vi "BCU参数读取-Auto.vi"(8 "CAN端口":u16(ring), 9 "设备索引号":u16(ring), 10 "CAN卡类型":u32(ring)=21, 11 "Myindex":dbl=1.0) -> (3 "成功":bool)   [LabVIEW 2013] (continued)
                    n501 = Greater Or Equal?(x=w675, y=30) -> (x >= y?=w673:bool)
                    n502 = Wait Until Next ms Multiple(millisecond multiple=u32 100 ("毫秒倍数")) -> ()  [unwired: 1 out]
                    n503 = Compound Arithmetic op=OR(w669, w670, w673) -> (w672:bool)
                  }
                }
                frame #4 {
                  n504 = call <vilib>:"Unset Busy.vi"() -> ()  [unwired: 2 in, 10 out]
                  n505 = case shown="假" w677 {
                    tunnel: w676 -> [w678 _]
                    frame False {
                      n506 = control-ref of="结果"() -> (w682:refnum<vi>)
                      n507 = Concatenate Strings(w678, "       写入失败" ("字符串")) -> (w681:string)
                      n508 = Build Array(w681) -> (w680:string[])
                      n509 = call "表格编辑.vi"("新元素/子数组"=w680, "活动单元格:单元格背景色"=u32 16740749, "MCListbox引用句柄"=w682) -> ()  [unwired: 9 out]
                    }
                    frame True {
                    }
                  }
                }
                frame #5 {
                  n510 = Increment(x=w688) -> (x+1=w684:i32)
                  n511 = Equal?(x=w689, y=w684) -> (x = y?=w687:bool)
                  n512 = And(x=w686, y=w687) -> (x .and. y?=w685:bool)
                  n513 = case shown="真" w685 {
                    frame False {
                    }
                    frame True {
                      n514 = control-ref of="结果"() -> (w693:refnum<vi>)
                      n515 = Concatenate Strings("写入完成" ("字符串")) -> (w692:string)
                      n516 = Build Array(w692) -> (w691:string[])
                      n517 = call "表格编辑.vi"("新元素/子数组"=w691, "活动单元格:单元格背景色"=u32 21937, "MCListbox引用句柄"=w693) -> ()  [unwired: 9 out]
                    }
                  }
                }
              }
            }
            n518 = local read "强制终止读写标记"() -> (w586:bool)
            n519 = Or(x=w584, y=w586) -> (x .or. y?=w585:bool)
          }
          n520 = stacked-sequence {
            tunnel: w576 -> [_]
            frame #0 {
              n521 = call <vilib>:"Unset Busy.vi"() -> ()  [unwired: 2 in, 10 out]
              n522 = local write "强制终止读写标记"(FALSE ("强制停止")) -> ()
            }
          }
        }
        frame "单个读取" {
          n523 = stacked-sequence {
            tunnel: [w726] -> w724
            frame #0 {
              n524 = local read "主从选择"() -> (w727:enum32{"主板", "从板"})
              n525 = case shown="\"主板\", 默认" w727 {
                tunnel: [w740 w823] -> w729
                tunnel: [w739 w824] -> w734
                tunnel: [0 ("从板号") w820] -> w733
                tunnel: [0 ("板号") u8 0 ("板号")] -> w732
                tunnel: [w735 w819] -> w730
                frame "主板", Default {
                  n526 = local read "主板选项"() -> (w736:string)
                  n527 = case shown="\"二维码\"" w736 {
                    tunnel: [_ u8[] [1, 2, 3, 4, 5, 6, 13, 8, 7, 9, 10, 11, 12] u8[] [1] u8[] [1] u8[] [1] u8[] [2] u8[] [3] u8[] [4] u8[] [5] u8[] [6] u8[] [13] u8[] [7] u8[] [8] u8[] [9] u8[] [10] u8[] [14] u8[] [11] u8[] [12] u8[] [2] u8[] [3] u8[] [1] u8[] [2] u8[] [1] u8[] [2] u8[] [3] u8[] [4] u8[] [1, 2, 3, 4]] -> w740
                    tunnel: [_ u8 128 ("命令") u8 129 ("命令") u8 128 ("命令") u8 140 ("命令") u8 128 ("命令") u8 128 ("命令") u8 128 ("命令") u8 128 ("命令") u8 128 ("命令") u8 128 ("命令") u8 128 ("命令") u8 128 ("命令") u8 128 ("命令") u8 128 ("命令") u8 128 ("命令") u8 128 ("命令") u8 128 ("命令") u8 129 ("命令") u8 129 ("命令") u8 130 ("命令") u8 130 ("命令") u8 132 ("命令") u8 132 ("命令") u8 132 ("命令") u8 132 ("命令") u8 132 ("命令")] -> w739
                    tunnel: [_ string[] ["产品编号", "电压个数", "通道电压数", "电压起始值", "温度个数", "温度起始值", "保险位置", "电池额定实际容量", "SOC", "配置文件版本", "参数修改记录", "车牌号", "SOH"] string[] ["一级故障阀值"] string[] ["产品编号"] string[] ["读二维码"] string[] ["电压个数"] string[] ["通道电压数"] string[] ["电压起始值"] string[] ["温度个数"] string[] ["温度起始值"] string[] ["保险位置"] string[] ["SOC"] string[] ["电池额定实际容量"] string[] ["配置文件版本"] string[] ["参数修改记录"] string[] ["校正时钟"] string[] ["车牌号"] string[] ["SOH"] string[] ["二级故障阀值"] string[] ["三级故障阀值"] string[] ["加热控制参数"] string[] ["充电控制参数"] string[] ["电池信息1"] string[] ["电池包组号"] string[] ["充放电安时"] string[] ["电池充放电次数"] string[] ["电池信息1", "电池包组号", "充放电安时", "电池充放电次数"]] -> w735
                    frame "假", Default {
                    }
                    frame "项目信息" {
                    }
                    frame "SOC过低", "SOC过高", "SOH过低", "充电电流过高", "单体电压过低", "单体电压过高", "单组电压不均衡", "单组温度不均衡", "放电电流过高", "极柱温度过高", "内阻过大", "温度过低", "温度过高", "一级故障阀值", "整组电压不均衡", "整组温度不均衡", "总电压过低", "总电压过高" {
                    }
                    frame "产品编号" {
                    }
                    frame "二维码" {
                    }
                    frame "电压个数" {
                    }
                    frame "通道电压数" {
                    }
                    frame "电压起始值" {
                    }
                    frame "温度个数" {
                    }
                    frame "温度起始值" {
                    }
                    frame "保险位置" {
                    }
                    frame "SOC" {
                    }
                    frame "电池额定实际容量" {
                    }
                    frame "配置文件版本" {
                    }
                    frame "参数修改记录" {
                    }
                    frame "校正时钟" {
                    }
                    frame "车牌号" {
                    }
                    frame "SOH" {
                    }
                    frame "SOC过低(2)", "SOC过高(2)", "SOH过低(2)", "充电电流过高(2)", "单体电压过低(2)", "单体电压过高(2)", "单组电压不均衡(2)", "单组温度不均衡(2)", "二级故障阀值", "放电电流过高(2)", "极柱温度过高(2)", "内阻过大(2)", "温度过低(2)", "温度过高(2)", "整组电压不均衡(2)", "整组温度不均衡(2)", "总电压过低(2)", "总电压过高(2)" {
                    }
                    frame "SOC过低(3)", "SOC过高(3)", "SOH过低(3)", "充电电流过高(3)", "单体电压过低(3)", "单体电压过高(3)", "单组电压不均衡(3)", "单组温度不均衡(3)", "放电电流过高(3)", "极柱温度过高(3)", "内阻过大(3)", "三级故障阀值", "温度过低(3)", "温度过高(3)", "整组电压不均衡(3)", "整组温度不均衡(3)", "总电压过低(3)", "总电压过高(3)" {
                    }
                    frame "风机关闭温差", "风机关闭温度", "风机开启温差", "风机开启温度", "加热关闭温差", "加热关闭温度", "加热开启温度", "加热控制参数" {
                    }
                    frame "充电控制参数", "电流步长", "最大允许充电电流", "最大允许充电温度", "最大允许单体电压", "最大允许总电压", "最小允许充电电流", "最小允许充电温度", "最小允许单体电压" {
                    }
                    frame "电池信息1" {
                    }
                    frame "电池包组号" {
                    }
                    frame "充放电安时" {
                    }
                    frame "电池充放电次数" {
                    }
                    frame "电池信息" {
                    }
                  }
                }
                frame "从板" {
                  n528 = local read "从板选项"() -> (w821:string)
                  n529 = case shown="\"二维码\"" w821 {
                    tunnel: [_ u8 0 ("命令") u8 10 ("命令") u8 0 ("命令") u8 0 ("命令") u8 0 ("命令") u8 0 ("命令") u8 0 ("命令") u8 0 ("命令") u8 2 ("命令") u8 2 ("命令") u8 2 ("命令") u8 3 ("命令") u8 6 ("命令") u8 6 ("命令") u8 6 ("命令") u8 3 ("命令") u8 3 ("命令") u8 3 ("命令") u8 3 ("命令") u8 3 ("命令") u8 3 ("命令") u8 3 ("命令")] -> w824
                    tunnel: [_ u8[] [6] u8[] [1] u8[] [6, 1, 2, 3, 4, 5] u8[] [1] u8[] [2] u8[] [3] u8[] [4] u8[] [5] u8[] [1] u8[] [2] u8[] [3] u8[] [1, 2, 3, 4, 5, 6, 7] u8[] [1, 2] u8[] [2] u8[] [1] u8[] [1] u8[] [2] u8[] [3] u8[] [4] u8[] [5] u8[] [6] u8[] [7]] -> w823
                    tunnel: [_ string[] ["从板号"] string[] ["读二维码"] string[] ["从板号", "电压起始值", "通道电压个数", "保险位置", "温度起始值", "加热控制参数"] string[] ["电压起始值"] string[] ["通道电压节数"] string[] ["保险位置"] string[] ["温度起始值"] string[] ["加热控制参数"] string[] ["一级故障阀值"] string[] ["二级故障阀值"] string[] ["三级故障阀值"] string[] ["电池包信息1", "电池包序号", "充放电安时", "充电次数时间", "SOC", "车牌号", "充电参数"] string[] ["均衡阀值", "充电结束电压"] string[] ["充电结束电压"] string[] ["均衡阀值"] string[] ["电池包信息1"] string[] ["电池包序号"] string[] ["充放电安时"] string[] ["充电次数时间"] string[] ["SOC"] string[] ["车牌号"] string[] ["充电参数"]] -> w819
                    frame "假", Default {
                    }
                    frame "从板号" {
                    }
                    frame "二维码" {
                    }
                    frame "从板信息" {
                    }
                    frame "电压个数" {
                    }
                    frame "通道电压节数" {
                    }
                    frame "保险位置" {
                    }
                    frame "温度个数" {
                    }
                    frame "风机关闭温差", "风机关闭温度", "风机开启温差", "风机开启温度", "加热关闭温差", "加热关闭温度", "加热开启温度", "加热控制参数" {
                    }
                    frame "SOC过低", "电压不均衡", "电压过低", "电压过高", "温度不均衡", "温度过低", "温度过高", "一级故障阀值" {
                    }
                    frame "SOC过低(2)", "电压不均衡(2)", "电压过低(2)", "电压过高(2)", "二级故障阀值", "温度不均衡(2)", "温度过低(2)", "温度过高(2)" {
                    }
                    frame "SOC过低(3)", "电压不均衡(3)", "电压过低(3)", "电压过高(3)", "三级故障阀值", "温度不均衡(3)", "温度过低(3)", "温度过高(3)" {
                    }
                    frame "快换参数" {
                    }
                    frame "均衡参数" {
                    }
                    frame "充电结束电压" {
                    }
                    frame "均衡阀值" {
                    }
                    frame "电池包信息1" {
                    }
                    frame "电池包序号" {
                    }
                    frame "充放电安时" {
                    }
                    frame "充电次数时间" {
                    }
                    frame "SOC" {
                    }
                    frame "车牌号" {
                    }
                    frame "充电参数" {
                    }
                  }
                  n530 = local read "从板号"() -> (w820:u8)
                }
              }
              n531 = Build Array(w732) -> (w731:i32[])
              n532 = local write "命令"(w734) -> ()
              n533 = Array Size(array=w729) -> (size(s)=w728:i32)
              n534 = for {
                tunnel: w729 -> [w899] mode=indexing
                tunnel: w734 -> [w898]
                tunnel: w733 -> [w897]
                tunnel: w731 -> [w896]
                tunnel: w730 -> [w895] mode=indexing
                tunnel: w728 -> [w894]
                tunnel: w727 -> [w892]
                tunnel: [w891] -> w726
                i -> [w893]
                n535 = while {
                  tunnel: w899 -> [w908]
                  tunnel: w898 -> [w907]
                  tunnel: w897 -> [w906]
                  tunnel: w896 -> [w905]
                  tunnel: w895 -> [w904]
                  tunnel: w894 -> [w903]
                  tunnel: w893 -> [w902]
                  tunnel: w892 -> [w901]
                  tunnel: [w900] -> w891
                  stop <- w900 stop-if-true
                  n536 = stacked-sequence {
                    seq-local: [_ _ _ _ w1058 _ _] -> [_ _ _ _ _ w1067 _]
                    tunnel: w908 -> [_ _ _ w1046 _ _ _]
                    tunnel: w907 -> [_ _ _ w1045 _ _ _]
                    tunnel: w906 -> [_ _ _ w1044 _ _ _]
                    tunnel: w905 -> [_ _ _ w1043 _ _ _]
                    tunnel: [_ _ _ _ w1059 _ _] -> w900
                    tunnel: w904 -> [w910 _ _ _ _ w1068 _]
                    tunnel: w903 -> [_ _ _ _ _ _ w1078]
                    tunnel: w902 -> [_ _ _ _ _ _ w1077]
                    tunnel: w901 -> [w909 _ _ _ _ _ _]
                    frame #0 {
                      n537 = case shown="\"从板\"" w909 {
                        tunnel: w910 -> [w911 w1003]
                        frame "主板", Default {
                          n538 = case shown="\"读二维码\"" w911 {
                            frame "假", Default {
                            }
                            frame "产品编号" {
                              n539 = control-ref of="产品编号"() -> (w913:refnum<vi>)
                              n540 = property class="Str"(reference=w913, "Value"="") -> ()  [unwired: 1 in, 2 out]
                            }
                            frame "读二维码" {
                              n541 = local write "二维码信息"("" ("二维码信息")) -> ()
                            }
                            frame "电压个数" {
                              n542 = local read "从板个数"() -> (w915:dbl)
                              n543 = control-ref of="项目信息"() -> (w919:refnum<vi>)
                              n544 = for {
                                N: w915 -> [_]
                                tunnel: [""] -> w918 mode=indexing
                              }
                              n545 = call "表格数据输入-8.6.vi"("行数"=u32 0, "列数"=u32 1, "字符串数组"=w918, "表格引用"=w919) -> ()  [unwired: 8 in]
                            }
                            frame "通道电压数" {
                              n546 = control-ref of="项目信息"() -> (w925:refnum<vi>)
                              n547 = for {
                                N: 20 -> [_]
                                tunnel: [""] -> w924 mode=indexing
                              }
                              n548 = local read "从板个数"() -> (w926:dbl)
                              n549 = Increment(x=w926) -> (x+1=w922:dbl)
                              n550 = call "表格数据输入-8.6.vi"("行数"=w922, "列数"=u32 1, "字符串数组"=w924, "表格引用"=w925) -> ()  [unwired: 8 in]
                            }
                            frame "电压起始值" {
                              n551 = local read "从板个数"() -> (w930:dbl)
                              n552 = Increment(x=w930) -> (x+1=w929:dbl)
                              n553 = control-ref of="项目信息"() -> (w936:refnum<vi>)
                              n554 = for {
                                N: w929 -> [_]
                                tunnel: [""] -> w935 mode=indexing
                              }
                              n555 = Multiply(x=u8 1, y=w930) -> (x*y=w932:dbl)
                              n556 = Add(x=w932, y=u8 21) -> (x+y=w928:dbl)
                              n557 = call "表格数据输入-8.6.vi"("行数"=w928, "列数"=u32 1, "字符串数组"=w935, "表格引用"=w936) -> ()  [unwired: 8 in]
                            }
                            frame "温度个数" {
                              n558 = local read "从板个数"() -> (w940:dbl)
                              n559 = Increment(x=w940) -> (x+1=w939:dbl)
                              n560 = control-ref of="项目信息"() -> (w946:refnum<vi>)
                              n561 = for {
                                N: w939 -> [_]
                                tunnel: [""] -> w945 mode=indexing
                              }
                              n562 = Multiply(x=u8 2, y=w940) -> (x*y=w942:dbl)
                              n563 = Add(x=w942, y=u8 22) -> (x+y=w938:dbl)
                              n564 = call "表格数据输入-8.6.vi"("行数"=w938, "列数"=u32 1, "字符串数组"=w945, "表格引用"=w946) -> ()  [unwired: 8 in]
                            }
                            frame "温度起始值" {
                              n565 = local read "从板个数"() -> (w950:dbl)
                              n566 = Increment(x=w950) -> (x+1=w949:dbl)
                              n567 = control-ref of="项目信息"() -> (w956:refnum<vi>)
                              n568 = for {
                                N: w949 -> [_]
                                tunnel: [""] -> w955 mode=indexing
                              }
                              n569 = Multiply(x=u8 3, y=w950) -> (x*y=w952:dbl)
                              n570 = Add(x=w952, y=u8 23) -> (x+y=w948:dbl)
                              n571 = call "表格数据输入-8.6.vi"("行数"=w948, "列数"=u32 1, "字符串数组"=w955, "表格引用"=w956) -> ()  [unwired: 8 in]
                            }
                            frame "保险位置" {
                              n572 = local read "从板个数"() -> (w960:dbl)
                              n573 = control-ref of="项目信息"() -> (w966:refnum<vi>)
                              n574 = for {
                                N: 10 -> [_]
                                tunnel: [""] -> w965 mode=indexing
                              }
                              n575 = Multiply(x=u8 4, y=w960) -> (x*y=w962:dbl)
                              n576 = Add(x=w962, y=u8 24) -> (x+y=w959:dbl)
                              n577 = call "表格数据输入-8.6.vi"("行数"=w959, "列数"=u32 1, "字符串数组"=w965, "表格引用"=w966) -> ()  [unwired: 8 in]
                            }
                            frame "电池额定实际容量" {
                              w968 = 0.0 ("值")
                              n578 = control-ref of="电池实际容量(A)"() -> (w969:refnum<vi>)
                              n579 = control-ref of="电池额定容量(A)"() -> (w970:refnum<vi>)
                              n580 = property class="DigNum (严格)"(reference=w969, "Value"=w968) -> ()  [unwired: 1 in, 2 out]
                              n581 = property class="DigNum (严格)"(reference=w970, "Value"=w968) -> ()  [unwired: 1 in, 2 out]
                            }
                            frame "SOC" {
                              n582 = control-ref of="SOC(%)"() -> (w971:refnum<vi>)
                              n583 = property class="DigNum (严格)"(reference=w971, "Value"=0.0 ("值")) -> ()  [unwired: 1 in, 2 out]
                            }
                            frame "配置文件版本" {
                              n584 = control-ref of="配置文件版本"() -> (w973:refnum<vi>)
                              n585 = property class="Str"(reference=w973, "Value"="" ("值")) -> ()  [unwired: 1 in, 2 out]
                            }
                            frame "参数修改记录" {
                              n586 = control-ref of="使用者"() -> (w976:refnum<vi>)
                              n587 = control-ref of="系统时钟"() -> (w977:refnum<vi>)
                              n588 = property class="DigNum (严格)"(reference=w976, "Value"=0.0 ("值")) -> ()  [unwired: 1 in, 2 out]
                              n589 = property class="Str"(reference=w977, "Value"="" ("值")) -> ()  [unwired: 1 in, 2 out]
                            }
                            frame "校正时钟" {
                              n590 = control-ref of="系统时钟"() -> (w979:refnum<vi>)
                              n591 = property class="Str"(reference=w979, "Value"="" ("值")) -> ()  [unwired: 1 in, 2 out]
                            }
                            frame "车牌号" {
                              n592 = control-ref of="车架(牌)号"() -> (w981:refnum<vi>)
                              n593 = property class="Str"(reference=w981, "Value"="" ("值")) -> ()  [unwired: 1 in, 2 out]
                            }
                            frame "SOH" {
                              n594 = control-ref of="SOH(%)"() -> (w984:refnum<vi>)
                              n595 = property class="DigNum (严格)"(reference=w984, "Value"=0.0 ("值")) -> ()  [unwired: 1 in, 2 out]
                            }
                            frame "一级故障阀值" {
                              n596 = local write "一级故障"(T10 {"总电压过高"=0.0, "整组电压不均衡"=0.0, "SOC过高"=0.0, "单体电压过高"=0.0, "总电压过低"=0.0, "温度过高"=0.0, "温度过低"=0.0, "单组电压不均衡"=0.0, "整组温度不均衡"=0.0, "单组温度不均衡"=0.0, "单体电压过低"=0.0, "充电电流过高"=0.0, "放电电流过高"=0.0, "SOC过低"=0.0, "内阻过大"=0.0, "极柱温度过高"=0.0, "SOH过低"=0.0} ("一级故障")) -> ()
                            }
                            frame "二级故障阀值" {
                              n597 = local write "一级故障 2"(T10 {"总电压过高"=0.0, "整组电压不均衡"=0.0, "SOC过高"=0.0, "单体电压过高"=0.0, "总电压过低"=0.0, "温度过高"=0.0, "温度过低"=0.0, "单组电压不均衡"=0.0, "整组温度不均衡"=0.0, "单组温度不均衡"=0.0, "单体电压过低"=0.0, "充电电流过高"=0.0, "放电电流过高"=0.0, "SOC过低"=0.0, "内阻过大"=0.0, "极柱温度过高"=0.0, "SOH过低"=0.0} ("一级故障")) -> ()
                            }
                            frame "三级故障阀值" {
                              n598 = local write "一级故障 3"(T10 {"总电压过高"=0.0, "整组电压不均衡"=0.0, "SOC过高"=0.0, "单体电压过高"=0.0, "总电压过低"=0.0, "温度过高"=0.0, "温度过低"=0.0, "单组电压不均衡"=0.0, "整组温度不均衡"=0.0, "单组温度不均衡"=0.0, "单体电压过低"=0.0, "充电电流过高"=0.0, "放电电流过高"=0.0, "SOC过低"=0.0, "内阻过大"=0.0, "极柱温度过高"=0.0, "SOH过低"=0.0} ("一级故障")) -> ()
                            }
                            frame "加热控制参数" {
                              n599 = local write "加热控制参数"(T11 {"风机开启温度"=0.0, "风机关闭温度"=0.0, "加热开启温度"=0.0, "加热关闭温度"=0.0, "风机开启温差"=0.0, "风机关闭温差"=0.0, "加热关闭温差"=0.0} ("加热控制参数")) -> ()
                            }
                            frame "充电控制参数" {
                              n600 = local write "一级故障 5"(T12 {"最大允许单体电压"=0.0, "最大允许总电压"=0.0, "最小允许单体电压"=0.0, "最大允许充电电流"=0.0, "最小允许充电电流"=0.0, "最大允许充电温度"=0.0, "最小允许充电温度"=0.0, "电流步长"=0.0} ("一级故障 5")) -> ()
                            }
                            frame "电池信息1" {
                              w990 = ""
                              w991 = 0.0 ("电池串联")
                              n601 = local read "电池信息"() -> (w993:T13)
                              n602 = Bundle By Name(cluster=w993, "电池串联"=w991, "电池并联"=w991, "电池包额定容量"=w991, "电池包额定能量(kWh)"=w991, "电池包额定总电压"=w991, "实际容量"=w991, "电池厂家"=w990, "电池类型"=w990, "电池生产日期"=w990) -> (w992:T13)
                              n603 = local write "电池信息"(w992) -> ()
                            }
                            frame "电池包组号" {
                              n604 = local read "电池信息"() -> (w996:T13)
                              n605 = Bundle By Name(cluster=w996, "电池包组号"="") -> (w995:T13)
                              n606 = local write "电池信息"(w995) -> ()
                            }
                            frame "充放电安时" {
                              w997 = 0.0 ("累计充电总安时")
                              n607 = local read "电池信息"() -> (w999:T13)
                              n608 = Bundle By Name(cluster=w999, "累计充电总安时"=w997, "累计放电总安时"=w997) -> (w998:T13)
                              n609 = local write "电池信息"(w998) -> ()
                            }
                            frame "电池充放电次数" {
                              w1000 = 0.0 ("累计充电总安时")
                              n610 = local read "电池信息"() -> (w1002:T13)
                              n611 = Bundle By Name(cluster=w1002, "电池充满次数"=w1000, "电池放空次数"=w1000, "电池充电次数"=w1000) -> (w1001:T13)
                              n612 = local write "电池信息"(w1001) -> ()
                            }
                          }
                        }
                        frame "从板" {
                          n613 = case shown="\"读二维码\"" w1003 {
                            frame "假", Default {
                            }
                            frame "电压起始值" {
                              n614 = control-ref of="项目信息 2"() -> (w1005:refnum<vi>)
                              n615 = for {
                                N: 1 -> [_]
                                tunnel: [""] -> w1008 mode=indexing
                              }
                              n616 = call "表格数据输入-8.6.vi"("行数"=u32 0, "列数"=u32 1, "字符串数组"=w1008, "表格引用"=w1005) -> ()  [unwired: 8 in]
                            }
                            frame "读二维码" {
                              n617 = local write "二维码信息 2"("" ("二维码信息 2")) -> ()
                            }
                            frame "通道电压节数" {
                              n618 = control-ref of="项目信息 2"() -> (w1011:refnum<vi>)
                              n619 = for {
                                N: 5 -> [_]
                                tunnel: [""] -> w1015 mode=indexing
                              }
                              n620 = call "表格数据输入-8.6.vi"("行数"=u32 22, "列数"=u32 1, "字符串数组"=w1015, "表格引用"=w1011) -> ()  [unwired: 8 in]
                            }
                            frame "保险位置" {
                              n621 = control-ref of="项目信息 2"() -> (w1017:refnum<vi>)
                              n622 = for {
                                N: 20 -> [_]
                                tunnel: [""] -> w1021 mode=indexing
                              }
                              n623 = call "表格数据输入-8.6.vi"("行数"=u32 2, "列数"=u32 1, "字符串数组"=w1021, "表格引用"=w1017) -> ()  [unwired: 8 in]
                            }
                            frame "温度起始值" {
                              n624 = control-ref of="项目信息 2"() -> (w1023:refnum<vi>)
                              n625 = for {
                                N: 1 -> [_]
                                tunnel: [""] -> w1027 mode=indexing
                              }
                              n626 = call "表格数据输入-8.6.vi"("行数"=u32 1, "列数"=u32 1, "字符串数组"=w1027, "表格引用"=w1023) -> ()  [unwired: 8 in]
                            }
                            frame "加热控制参数" {
                              n627 = local write "加热控制参数"(T11 {"风机开启温度"=0.0, "风机关闭温度"=0.0, "加热开启温度"=0.0, "加热关闭温度"=0.0, "风机开启温差"=0.0, "风机关闭温差"=0.0, "加热关闭温差"=0.0} ("加热控制参数")) -> ()
                            }
                            frame "一级故障阀值" {
                              n628 = local write "一级故障 6"(T15 {"电压过高"=0.0, "电压过低"=0.0, "温度过高"=0.0, "温度过低"=0.0, "电压不均衡(V)"=0.0, "温度不均衡"=0.0, "SOC过低"=0.0} ("一级故障 6")) -> ()
                            }
                            frame "二级故障阀值" {
                              n629 = local write "一级故障 7"(T15 {"电压过高"=0.0, "电压过低"=0.0, "温度过高"=0.0, "温度过低"=0.0, "电压不均衡(V)"=0.0, "温度不均衡"=0.0, "SOC过低"=0.0} ("一级故障 7")) -> ()
                            }
                            frame "三级故障阀值" {
                              n630 = local write "一级故障 8"(T15 {"电压过高"=0.0, "电压过低"=0.0, "温度过高"=0.0, "温度过低"=0.0, "电压不均衡(V)"=0.0, "温度不均衡"=0.0, "SOC过低"=0.0} ("一级故障 7")) -> ()
                            }
                            frame "均衡参数" {
                              n631 = local write "均衡参数"(T17 {"充电结束电压(90%)"=0.0, "充电结束电压(91%)"=0.0, "充电结束电压(92%)"=0.0, "充电结束电压(93%)"=0.0, "充电结束电压(94%)"=0.0, "均衡计算-电压高阀值1级"=0.0, "均衡计算-电压高阀值2级"=0.0, "均衡计算-电压低阀值1级"=0.0, "均衡计算-电压低阀值2级"=0.0, "均衡计算-最低电压阀值"=0.0, "均衡停止-最低电压阀值"=0.0, "均衡计算-电压极差阀值"=0.0, "充电结束电压(95%)"=0.0, "充电结束电压(96%)"=0.0, "充电结束电压(97%)"=0.0, "充电结束电压(98%)"=0.0, "充电结束电压(99%)"=0.0, "充电结束电压(100%)"=0.0} ("均衡参数")) -> ()
                            }
                            frame "均衡阀值" {
                              w1034 = sgl 0.0 ("均衡计算-电压高阀值1级")
                              n632 = local read "均衡参数"() -> (w1035:T17)
                              n633 = Bundle By Name(cluster=w1035, "均衡计算-电压高阀值1级"=w1034, "均衡计算-电压高阀值2级"=w1034, "均衡计算-电压低阀值1级"=w1034, "均衡计算-电压低阀值2级"=w1034, "均衡计算-最低电压阀值"=w1034, "均衡停止-最低电压阀值"=w1034, "均衡计算-电压极差阀值"=w1034) -> (w1036:T17)
                              n634 = local write "均衡参数"(w1036) -> ()
                            }
                            frame "充电结束电压" {
                              w1037 = sgl 0.0 ("均衡计算-电压高阀值1级")
                              n635 = local read "均衡参数"() -> (w1038:T17)
                              n636 = Bundle By Name(cluster=w1038, "充电结束电压(90%)"=w1037, "充电结束电压(91%)"=w1037, "充电结束电压(92%)"=w1037, "充电结束电压(93%)"=w1037, "充电结束电压(94%)"=w1037, "充电结束电压(95%)"=w1037, "充电结束电压(96%)"=w1037, "充电结束电压(97%)"=w1037, "充电结束电压(98%)"=w1037, "充电结束电压(99%)"=w1037, "充电结束电压(100%)"=w1037) -> (w1039:T17)
                              n637 = local write "均衡参数"(w1039) -> ()
                            }
                          }
                        }
                      }
                    }
                    frame #1 {
                      w1040 = FALSE ("流控帧")
                      w1041 = TRUE ("流控帧 2")
                      n638 = global write "EV05全局变量1.vi" "写入超时"(w1040) -> ()
                      n639 = global write "EV05全局变量1.vi" "流控帧"(w1040) -> ()
                      n640 = local write "写?"(w1040) -> ()
                      n641 = call <vilib>:"Set Busy.vi"("disable click? (T)"=w1040) -> ()  [unwired: 3 in, 8 out]
                      n642 = local write "消除"(w1041) -> ()
                      n643 = local write "控制1"(w1041) -> ()
                      n644 = global write "EV05全局变量1.vi" "流控帧 2"(w1041) -> ()
                    }
                    frame #2 {
                      n645 = Wait Until Next ms Multiple(millisecond multiple=u32 150 ("毫秒倍数")) -> ()  [unwired: 1 out]
                    }
                    frame #3 {
                      n646 = local read "设备索引号"() -> (w1048:u16)
                      n647 = local read "CAN卡类型"() -> (w1049:u32)
                      n648 = local read "CAN端口"() -> (w1047:u16)
                      n649 = stacked-sequence {
                        tunnel: w1049 -> [_ w1057]
                        tunnel: w1048 -> [_ w1056]
                        tunnel: w1047 -> [_ w1055]
                        tunnel: w1046 -> [_ w1054]
                        tunnel: w1045 -> [_ w1053]
                        tunnel: w1044 -> [_ w1052]
                        tunnel: w1043 -> [_ w1051]
                        frame #0 {
                        }
                        frame #1 {
                          n650 = call "多帧发送机制(EV05).vi"("can卡类型"=w1057, "设备索引号"=w1056, "CAN端口"=w1055, "命令"=w1053, "板号"=w1052, "命令序号"=w1054, "输入数据"=w1051) -> ("错误输出"=w1050:errorcluster)  [unwired: 2 in, 10 out]
                          n651 = call <vilib>:"Clear Errors.vi"("error in (no error)"=w1050) -> ()  [unwired: 6 in, 1 out]
                        }
                      }
                      "命令序号" <- w1046
                    }
                    frame #4 {
                      n652 = while {
                        tunnel: [w1062] -> w1059
                        tunnel: [w1061] -> w1058
                        i -> [w1065]
                        stop <- w1062 stop-if-true
                        n653 = local read "强制终止读写标记"() -> (w1060:bool)
                        n654 = global read "EV05全局变量1.vi" "写入超时"() -> (w1061:bool)
                        n655 = Greater Or Equal?(x=w1065, y=30) -> (x >= y?=w1063:bool)
                        n656 = Compound Arithmetic op=OR(w1060, w1061, w1063) -> (w1062:bool)
                        n657 = Wait Until Next ms Multiple(millisecond multiple=u32 100 ("毫秒倍数")) -> ()  [unwired: 1 out]
                      }
                    }
                    frame #5 {
                      n658 = case shown="假" w1067 {
                        tunnel: w1068 -> [w1071 _]
                        frame False {
                          n659 = control-ref of="结果"() -> (w1070:refnum<vi>)
                          n660 = Concatenate Strings(w1071, "     读取失败" ("字符串")) -> (w1073:string)
                          n661 = Build Array(w1073) -> (w1069:string[])
                          n662 = call "表格编辑.vi"("新元素/子数组"=w1069, "活动单元格:单元格背景色"=u32 16740749, "MCListbox引用句柄"=w1070) -> ()  [unwired: 9 out]
                        }
                        frame True {
                        }
                      }
                    }
                    frame #6 {
                      n663 = Increment(x=w1077) -> (x+1=w1076:i32)
                      n664 = Equal?(x=w1078, y=w1076) -> (x = y?=w1075:bool)
                      n665 = case shown="真" w1075 {
                        frame False {
                        }
                        frame True {
                          n666 = control-ref of="结果"() -> (w1080:refnum<vi>)
                          n667 = Concatenate Strings("读取完成" ("字符串")) -> (w1082:string)
                          n668 = Build Array(w1082) -> (w1079:string[])
                          n669 = call "表格编辑.vi"("新元素/子数组"=w1079, "活动单元格:单元格背景色"=u32 21937, "MCListbox引用句柄"=w1080) -> ()  [unwired: 9 out]
                        }
                      }
                    }
                  }
                }
              }
            }
          }
          n670 = stacked-sequence {
            tunnel: w724 -> [_]
            frame #0 {
              n671 = call <vilib>:"Unset Busy.vi"() -> ()  [unwired: 11 in, 1 out]
              n672 = local write "强制终止读写标记"(FALSE ("强制停止")) -> ()
            }
          }
        }
        frame "全部读取" {
          n673 = stacked-sequence {
            seq-local: [w1089 _ _ _] -> [_ _ _ w2072]
            seq-local: [w1088 _ _ _] -> [_ _ _ _]
            tunnel: [_ _ w1701 _] -> w1086
            tunnel: w1084 -> [_ w1289 _ _]
            frame #0 {
              n674 = local read "主从选择"() -> (w1089:enum32{"主板", "从板"})
              n675 = local read "路径"() -> (w1090:path)
              n676 = Empty String/Path?(string/path=w1090) -> (empty?=w1088:bool)
              n677 = disable-structure shown="禁用" {
                disable-tunnel: w1090 -> [w1093 _]
                disable-tunnel: w1088 -> [w1092 _]
                disable-tunnel: w1089 -> [w1091 _]
                frame Disabled {
                  n678 = case shown="假" w1092 {
                    tunnel: w1093 -> [w1097 _]
                    tunnel: w1091 -> [w1096 _]
                    frame False {
                      n679 = control-ref of="结果"() -> (w1094:refnum<vi>)
                      n680 = call-poly <vilib>:"Read From Spreadsheet File.vi"("file path (dialog if empty)"=w1097) -> ("all rows"=w1095:string[][])  [unwired: 3 in, 7 out]
                      n681 = case shown="\"主板\", 默认" w1096 {
                        tunnel: w1095 -> [w1099 w1194]
                        tunnel: w1094 -> [w1098 w1193]
                        frame "主板", Default {
                          n682 = stacked-sequence {
                            tunnel: w1099 -> [w1108 w1132 w1189]
                            tunnel: w1098 -> [w1105 _ w1160]
                            frame #0 {
                              n683 = Index Array(array=w1108, index (col)=3 ("禁用的索引 (列)")) -> (element=w1122:string[])  [unwired: 1 in]
                              n684 = Index Array(array=w1108, index (col)=1 ("禁用的索引 (列)")) -> (element=w1128:string[])  [unwired: 1 in]
                              n685 = Delete From Array(array=w1122, length=4 ("长度"), index=0 ("索引")) -> (deleted portion=w1119:string[], array with subset deleted=w1113:string[])
                              n686 = Delete From Array(array=w1128, length=1 ("长度"), index=0 ("索引")) -> (deleted portion=w1125:string[], array with subset deleted=w1102:string[])
                              n687 = Build Array("正在读取主板配置文件...") -> (w1106:string[])
                              n688 = Index Array(array=w1113) -> (element #1=w1112:string, element #2=w1111:string, element #3=w1110:string, element #4=w1109:string)  [unwired: 4 in]
                              n689 = for {
                                tunnel: w1119 -> [w1131] mode=indexing
                                tunnel: [w1130] -> w1118 mode=indexing
                                n690 = Fract/Exp String To Number(string=w1131) -> (number=w1130:dbl)  [unwired: 4 out]
                              }
                              n691 = Index Array(array=w1125) -> (element=w1124:string)  [unwired: 1 in]
                              n692 = global write "读配置文件全局.vi" "表格输入"(w1102) -> ()
                              n693 = call "表格编辑.vi"("新元素/子数组"=w1106, "活动单元格:单元格背景色"=u32 6618880, "MCListbox引用句柄"=w1105) -> ()  [unwired: 9 out]
                              n694 = Decimal String To Number(string=w1124) -> (number=w1103:i32)  [unwired: 1 in, 2 out]
                              n695 = global read "读配置文件全局.vi" "项目信息"() -> (w1101:T22)
                              n696 = Index Array(array=w1118) -> (element #1=w1117:dbl, element #2=w1116:dbl, element #3=w1115:dbl, element #4=w1114:dbl)  [unwired: 4 in]
                              n697 = global write "读配置文件全局.vi" "从板个数"(w1103) -> ()
                              n698 = Bundle(cluster=w1101, "电池额定容量"=w1117, "电池实际容量"=w1116, "车牌号"=w1112, "配置文件版本"=w1111, "SOH"=w1114, "SOC"=w1115, "产品编号"=w1110, "系统时钟"=w1109) -> (w1100:T22)  [unwired: 1 out]
                              n699 = global write "读配置文件全局.vi" "项目信息"(w1100) -> ()
                            }
                            frame #1 {
                              n700 = Index Array(array=w1132, index (col)=3 ("禁用的索引 (列)")) -> (element=w1150:string[])  [unwired: 1 in]
                              n701 = Index Array(array=w1132, index (col)=5 ("禁用的索引 (列)")) -> (element=w1144:string[])  [unwired: 1 in]
                              n702 = for {
                                tunnel: w1144 -> [w1157] mode=indexing
                                tunnel: [w1156] -> w1143 mode=indexing
                                n703 = Fract/Exp String To Number(string=w1157) -> (number=w1156:dbl)  [unwired: 4 out]
                              }
                              n704 = Delete From Array(array=w1150, length=17 ("长度"), index=8 ("索引")) -> (deleted portion=w1148:string[])  [unwired: 1 out]
                              n705 = for {
                                tunnel: w1148 -> [w1159] mode=indexing
                                tunnel: [w1158] -> w1146 mode=indexing
                                n706 = Fract/Exp String To Number(string=w1159) -> (number=w1158:dbl)  [unwired: 4 out]
                              }
                              n707 = global write "读配置文件全局.vi" "二级故障"(w1143) -> ()
                              n708 = global write "读配置文件全局.vi" "一级故障"(w1146) -> ()
                              n709 = Index Array(array=w1132, index (col)=7 ("禁用的索引 (列)")) -> (element=w1141:string[])  [unwired: 1 in]
                              n710 = Index Array(array=w1132, index (col)=9 ("禁用的索引 (列)")) -> (element=w1138:string[])  [unwired: 1 in]
                              n711 = for {
                                tunnel: w1141 -> [w1155] mode=indexing
                                tunnel: [w1154] -> w1140 mode=indexing
                                n712 = Fract/Exp String To Number(string=w1155) -> (number=w1154:dbl)  [unwired: 4 out]
                              }
                              n713 = for {
                                tunnel: w1138 -> [w1153] mode=indexing
                                tunnel: [w1152] -> w1137 mode=indexing
                                n714 = Fract/Exp String To Number(string=w1153) -> (number=w1152:dbl)  [unwired: 4 out]
                              }
                              n715 = Delete From Array(array=w1137, length=6 ("长度"), index=0 ("索引")) -> (deleted portion=w1134:dbl[], array with subset deleted=w1133:dbl[])
                              n716 = global write "读配置文件全局.vi" "三级故障"(w1140) -> ()
                              n717 = global write "读配置文件全局.vi" "加热控制参数"(w1134) -> ()
                              n718 = global write "读配置文件全局.vi" "充电控制参数"(w1133) -> ()
                            }
                            frame #2 {
                              n719 = call <vilib>:"Unset Busy.vi"() -> ()  [unwired: 2 in, 10 out]
                              n720 = Index Array(array=w1189, index (col)=11 ("禁用的索引 (列)")) -> (element=w1186:string[])  [unwired: 1 in]
                              n721 = Delete From Array(array=w1186, length=6 ("长度"), index=0 ("索引")) -> (deleted portion=w1168:string[], array with subset deleted=w1167:string[])
                              n722 = for {
                                tunnel: w1167 -> [w1192] mode=indexing
                                tunnel: [w1191] -> w1185 mode=indexing
                                n723 = Fract/Exp String To Number(string=w1192) -> (number=w1191:dbl)  [unwired: 4 out]
                              }
                              n724 = Index Array(array=w1168) -> (element #1=w1184:string, element #2=w1183:string, element #3=w1182:string, element #4=w1181:string, element #5=w1180:string, element #6=w1179:string)  [unwired: 6 in]
                              n725 = Index Array(array=w1185) -> (element #1=w1178:dbl, element #2=w1177:dbl, element #3=w1176:dbl, element #4=w1175:dbl, element #5=w1174:dbl, element #6=w1173:dbl, element #7=w1172:dbl, element #8=w1171:dbl, element #9=w1170:dbl, element #10=w1169:dbl, element #11=w1164:dbl)  [unwired: 11 in]
                              n726 = global read "读配置文件全局.vi" "电池信息"() -> (w1166:T23)
                              n727 = Build Array("配置文件读取完成") -> (w1162:string[])
                              n728 = Bundle(cluster=w1166, "电池串联"=w1178, "电池并联"=w1177, "累计放电总安时"=w1175, "电池包额定容量"=w1174, "电池包额定能量"=w1173, "电池包额定总电压"=w1172, "累计充电总安时"=w1176, "电池充满次数"=w1171, "电池放空次数"=w1170, "电池充电次数"=w1169, "电池生产日期"=w1184, "电池厂家"=w1183, "电池类型"=w1182, "电池包组号"=w1181, "电池包产权标识"=w1180, "电池应用车型"=w1179, "实际容量"=w1164) -> (w1165:T23)
                              n729 = call "表格编辑.vi"("新元素/子数组"=w1162, "活动单元格:单元格背景色"=u32 6618880, "MCListbox引用句柄"=w1160) -> ()  [unwired: 9 out]
                              n730 = global write "读配置文件全局.vi" "电池信息"(w1165) -> ()
                            }
                          }
                        }
                        frame "从板" {
                          n731 = stacked-sequence {
                            tunnel: w1194 -> [w1202 w1230 w1274]
                            tunnel: w1193 -> [w1199 _ w1250]
                            frame #0 {
                              n732 = Index Array(array=w1202, index (col)=1 ("禁用的索引 (列)")) -> (element=w1212:string[])  [unwired: 1 in]
                              n733 = Index Array(array=w1202, index (col)=3 ("禁用的索引 (列)")) -> (element=w1206:string[])  [unwired: 1 in]
                              n734 = Delete From Array(array=w1212, length=1 ("长度"), index=0 ("索引")) -> (deleted portion=w1209:string[], array with subset deleted=w1196:string[])
                              n735 = Delete From Array(array=w1206, length=6 ("长度"), index=0 ("索引")) -> (deleted portion=w1203:string[])  [unwired: 1 out]
                              n736 = for {
                                tunnel: w1203 -> [w1215] mode=indexing
                                tunnel: [w1214] -> w1195 mode=indexing
                                i -> [w1216]
                                n737 = Fract/Exp String To Number(string=w1215, default (0 dbl)=w1216) -> (number=w1214:i32)  [unwired: 3 out]
                              }
                              n738 = Index Array(array=w1209) -> (element=w1208:string)  [unwired: 1 in]
                              n739 = global write "读配置文件全局2.vi" "表格"(w1196) -> ()
                              n740 = Build Array("正在读取从板配置文件...") -> (w1200:string[])
                              n741 = Decimal String To Number(string=w1208) -> (number=w1197:i32)  [unwired: 1 in, 2 out]
                              n742 = call "表格编辑.vi"("新元素/子数组"=w1200, "活动单元格:单元格背景色"=u32 6618880, "MCListbox引用句柄"=w1199) -> ()  [unwired: 9 out]
                              n743 = global write "读配置文件全局2.vi" "加热控制参数"(w1195) -> ()
                              n744 = global write "读配置文件全局2.vi" "从板板号"(w1197) -> ()
                            }
                            frame #1 {
                              n745 = Index Array(array=w1230, index (col)=3 ("禁用的索引 (列)")) -> (element=w1220:string[])  [unwired: 1 in]
                              n746 = Array Subset(array=w1220, index=6 ("索引"), length=7 ("长度")) -> (w1227:string[])
                              n747 = Array Subset(array=w1220, index=13 ("索引"), length=7 ("长度")) -> (w1226:string[])
                              n748 = Array Subset(array=w1220, index=20 ("索引"), length=7 ("长度")) -> (w1221:string[])
                              n749 = for {
                                tunnel: w1227 -> [w1237] mode=indexing
                                tunnel: [w1236] -> w1217 mode=indexing
                                n750 = Fract/Exp String To Number(string=w1237) -> (number=w1236:dbl)  [unwired: 4 out]
                              }
                              n751 = for {
                                tunnel: w1226 -> [w1235] mode=indexing
                                tunnel: [w1234] -> w1218 mode=indexing
                                n752 = Fract/Exp String To Number(string=w1235) -> (number=w1234:dbl)  [unwired: 4 out]
                              }
                              n753 = for {
                                tunnel: w1221 -> [w1233] mode=indexing
                                tunnel: [w1232] -> w1219 mode=indexing
                                n754 = Fract/Exp String To Number(string=w1233) -> (number=w1232:dbl)  [unwired: 4 out]
                              }
                              n755 = global write "读配置文件全局2.vi" "一级故障阀值"(w1217) -> ()
                              n756 = global write "读配置文件全局2.vi" "二级故障阀值"(w1218) -> ()
                              n757 = global write "读配置文件全局2.vi" "三级故障阀值"(w1219) -> ()
                            }
                            frame #2 {
                              n758 = Index Array(array=w1274, index (col)=5 ("禁用的索引 (列)")) -> (element=w1272:string[])  [unwired: 1 in]
                              n759 = Delete From Array(array=w1272, length=1 ("长度"), index=16 ("索引")) -> (deleted portion=w1268:string[], array with subset deleted=w1269:string[])
                              n760 = for {
                                tunnel: w1269 -> [w1277] mode=indexing
                                tunnel: [w1276] -> w1273 mode=indexing
                                n761 = Fract/Exp String To Number(string=w1277) -> (number=w1276:dbl)  [unwired: 4 out]
                              }
                              n762 = Index Array(array=w1273) -> (element #1=w1267:dbl, element #2=w1266:dbl, element #3=w1265:dbl, element #4=w1264:dbl, element #5=w1263:dbl, element #6=w1262:dbl, element #7=w1261:dbl, element #8=w1260:dbl, element #9=w1259:dbl, element #10=w1258:dbl, element #11=w1257:dbl, element #12=w1248:dbl, element #13=w1256:dbl, element #14=w1255:dbl, element #15=w1254:dbl, element #16=w1253:dbl, element #17=w1246:dbl, element #18=w1245:dbl, element #19=w1244:dbl, element #20=w1243:dbl, element #21=w1242:dbl, element #22=w1241:dbl)  [unwired: 22 in]
                              n763 = Build Array("配置文件读取完成") -> (w1251:string[])
                              n764 = Index Array(array=w1268, index=22 ("索引")) -> (element=w1247:string)
                              n765 = global read "读配置文件全局2.vi" "电池组信息"() -> (w1239:T24)
                              n766 = call "表格编辑.vi"("新元素/子数组"=w1251, "活动单元格:单元格背景色"=u32 6618880, "MCListbox引用句柄"=w1250) -> ()  [unwired: 9 out]
                              n767 = Bundle(cluster=w1239, "电池类型"=w1267, "电池厂家"=w1266, "电池地区"=w1265, "电池组序号"=w1264, "电池包串联数"=w1263, "电池包并联数"=w1262, "电池包安时数"=w1261, "电池包序号"=w1260, "充电次数"=w1259, "充满电时间"=w1258, "放空时间"=w1257, "车牌号"=w1247, "最大允许单体电压"=w1248, "最大允许总电压"=w1256, "最大允许温度"=w1255, "最小允许温度"=w1254, "最大允许充电电流"=w1253, "最小允许充电电流"=w1246, "最小允许单体电压"=w1245, "电流步长"=w1244, "SOC"=w1243, "充电总安时"=w1242, "放电总这时"=w1241) -> (w1238:T24)
                              n768 = call <vilib>:"Unset Busy.vi"() -> ()  [unwired: 2 in, 10 out]
                              n769 = global write "读配置文件全局2.vi" "电池组信息"(w1238) -> ()
                            }
                          }
                        }
                      }
                    }
                    frame True {
                    }
                  }
                }
                frame Enabled {
                }
              }
              n770 = case shown="\"主板\", 默认" w1089 {
                frame "主板", Default {
                  w1278 = FALSE
                  n771 = global write "读配置文件全局.vi" "SOC判定"(w1278) -> ()
                  n772 = global write "读配置文件全局.vi" "SOH判定"(w1278) -> ()
                  n773 = global write "读配置文件全局.vi" "车牌号判定"(w1278) -> ()
                  n774 = global write "读配置文件全局.vi" "电池信息1判定"(w1278) -> ()
                  n775 = global write "读配置文件全局.vi" "保险位置判定"(w1278) -> ()
                  n776 = global write "读配置文件全局.vi" "产品编号判定"(w1278) -> ()
                  n777 = global write "读配置文件全局.vi" "充放电安时判定"(w1278) -> ()
                  n778 = global write "读配置文件全局.vi" "从板个数判定"(w1278) -> ()
                  n779 = global write "读配置文件全局.vi" "电池包组号判定"(w1278) -> ()
                  n780 = global write "读配置文件全局.vi" "电压个数判定"(w1278) -> ()
                  n781 = global write "读配置文件全局.vi" "电压起始值判定"(w1278) -> ()
                  n782 = global write "读配置文件全局.vi" "充电控制参数判定"(w1278) -> ()
                  n783 = global write "读配置文件全局.vi" "电池充放电次数判定"(w1278) -> ()
                  n784 = global write "读配置文件全局.vi" "电池额定实际容量判定"(w1278) -> ()
                  n785 = global write "读配置文件全局.vi" "二级故障判定"(w1278) -> ()
                  n786 = global write "读配置文件全局.vi" "三级故障判定"(w1278) -> ()
                  n787 = global write "读配置文件全局.vi" "通道电压数判定"(w1278) -> ()
                  n788 = global write "读配置文件全局.vi" "温度个数判定"(w1278) -> ()
                  n789 = global write "读配置文件全局.vi" "一级故障判定"(w1278) -> ()
                  n790 = global write "读配置文件全局.vi" "温度起始值判定"(w1278) -> ()
                  n791 = global write "读配置文件全局.vi" "加热控制参数判定"(w1278) -> ()
                  n792 = global write "读配置文件全局.vi" "配置文件版本判定"(w1278) -> ()
                }
                frame "从板" {
                  w1279 = FALSE
                  n793 = disable-structure shown="禁用" {
                    frame Disabled {
                      n794 = global read "读配置文件全局2.vi" "充电次数时间判定"() -> ()  [unwired: 1 in]
                      n795 = global read "读配置文件全局2.vi" "电池包信息1判定"() -> ()  [unwired: 1 in]
                      n796 = global read "读配置文件全局2.vi" "电池包序号判定"() -> ()  [unwired: 1 in]
                      n797 = global read "读配置文件全局2.vi" "充放电安时判定"() -> ()  [unwired: 1 in]
                      n798 = global read "读配置文件全局2.vi" "车牌号判定"() -> ()  [unwired: 1 in]
                      n799 = global read "读配置文件全局2.vi" "充电参数判定"() -> ()  [unwired: 1 in]
                      n800 = global read "读配置文件全局2.vi" "保险位置判定"() -> ()  [unwired: 1 in]
                    }
                    frame Enabled {
                    }
                  }
                  n801 = global write "读配置文件全局2.vi" "从板号判定"(w1279) -> ()
                  n802 = global write "读配置文件全局2.vi" "通道电压判定"(w1279) -> ()
                  n803 = global write "读配置文件全局2.vi" "保险位置判定"(w1279) -> ()
                  n804 = global write "读配置文件全局2.vi" "二级故障判定"(w1279) -> ()
                  n805 = global write "读配置文件全局2.vi" "三级故障判定"(w1279) -> ()
                  n806 = global write "读配置文件全局2.vi" "电压起始值判定"(w1279) -> ()
                  n807 = global write "读配置文件全局2.vi" "温度起始值判定"(w1279) -> ()
                  n808 = global write "读配置文件全局2.vi" "一级故障判定"(w1279) -> ()
                }
              }
            }
            frame #1 {
              n809 = call <vilib>:"Open Config Data.vi"("error in (no error)"=w1289, "create file if necessary (T)"=FALSE, "configuration file path"=path "D:/自动测试项目文件/ProjectSetting.ini") -> ("error out"=w1288:errorcluster, "refnum"=w1291:T25)  [unwired: 6 in, 1 out]
              n810 = call-poly <vilib>:"Read Key.vi"("section"="PROJECT", "error in (no error)"=w1288, "key"="配置文件", "refnum"=w1291) -> ("error out"=w1283:errorcluster, "value"=w1281:string, "refnum out"=w1284:T25)  [unwired: 4 in, 1 out]
              n811 = call <vilib>:"Close Config Data.vi"("error in (no error)"=w1283, "refnum"=w1284) -> ()  [unwired: 8 in, 2 out]
              n812 = Build Path(base path=path "D:/自动测试项目文件" ("configuration file path"), name or relative path=w1281) -> (appended path=w1280:path)
              n813 = Strip Path(path=w1280) -> (stripped path=w1292:path, name=w1299:string)
              n814 = Match Pattern(string=w1299, regular expression=".ini" ("正则表达式")) -> (offset past match=w1297:i32)  [unwired: 1 in, 3 out]
              n815 = Not Equal?(x=w1297, y=-1) -> (x != y?=w1293:bool)
              n816 = case shown="真" w1293 {
                tunnel: w1280 -> [_ w1309]
                tunnel: [_ w1318] -> w1294
                frame False {
                }
                frame True {
                  w1321 = "MD5码" ("key")
                  w1322 = "总信息" ("section")
                  n817 = Strip Path(path=w1309) -> (stripped path=w1307:path, name=w1306:string)
                  n818 = Match Pattern(string=w1306, regular expression=".ini" ("正则表达式")) -> (before substring=w1303:string, match substring=w1304:string)  [unwired: 1 in, 2 out]
                  n819 = Concatenate Strings(w1303, "-rc" ("字符串"), w1304) -> (w1302:string)
                  n820 = Build Path(base path=w1307, name or relative path=w1302) -> (appended path=w1308:path)
                  n821 = Copy(10:w1308, 11:w1309) -> (3:w1313:path)  [unwired: 3 in, 2 out]
                  n822 = call <vilib>:"Open Config Data.vi"("create file if necessary (T)"=FALSE, "configuration file path"=w1313) -> ("refnum"=w1324:T25)  [unwired: 7 in, 2 out]
                  n823 = call-poly <vilib>:"Read Key.vi"("section"=w1322, "key"=w1321, "refnum"=w1324) -> ("value"=w1319:string, "refnum out"=w1323:T25)  [unwired: 5 in, 2 out]
                  n824 = call-poly <vilib>:"Write Key.vi"("section"=w1322, "value"=w1321, "key"=w1321, "refnum"=w1323) -> ("error out"=w1317:errorcluster, "found?"=w1316:bool, "refnum out"=w1315:T25)  [unwired: 5 in]
                  n825 = call <vilib>:"Close Config Data.vi"("error in (no error)"=w1317, "write file if changed (T)"=w1316, "refnum"=w1315) -> ("error out"=w1314:errorcluster, "file path"=w1311:path)  [unwired: 7 in]
                  n826 = call <vilib>:"MD5Checksum File.vi"("error in (no error)"=w1314, "Path"=w1311) -> ("error out"=w1312:errorcluster, "MD5 message-digest"=w1320:string)  [unwired: 8 in]
                  n827 = Equal?(x=w1320, y=w1319) -> (x = y?=w1318:bool)
                  n828 = Delete(path (use dialog)=w1311, error in=w1312) -> (error out=w1310:errorcluster)  [unwired: 3 in, 2 out]
                  n829 = call <vilib>:"Clear Errors.vi"("error in (no error)"=w1310) -> ()  [unwired: 6 in, 1 out]
                }
              }
              n830 = global write "配置文件全局.vi" "诊断标定读取地址"(w1292) -> ()
              n831 = And(x=w1293, y=w1294) -> (x .and. y?=w1295:bool)
              n832 = control-ref of="结果"() -> (w1300:refnum<vi>)
              n833 = case shown="假" w1295 {
                tunnel: w1280 -> [_ w1342]
                tunnel: w1300 -> [w1328 w1341]
                tunnel: w1294 -> [w1327 _]
                tunnel: w1293 -> [w1326 _]
                frame False {
                  n834 = stacked-sequence {
                    tunnel: w1326 -> [w1330 _]
                    tunnel: w1328 -> [w1329 w1336]
                    tunnel: w1327 -> [_ w1335]
                    frame #0 {
                      n835 = case shown="假" w1330 {
                        tunnel: w1329 -> [w1332 _]
                        frame False {
                          n836 = Build Array("文件格式错误") -> (w1333:string[])
                          n837 = call "表格编辑.vi"("新元素/子数组"=w1333, "活动单元格:单元格背景色"=u32 16711680, "MCListbox引用句柄"=w1332) -> ()  [unwired: 9 out]
                        }
                        frame True {
                        }
                      }
                    }
                    frame #1 {
                      n838 = case shown="假" w1335 {
                        tunnel: w1336 -> [w1338 _]
                        frame False {
                          n839 = Build Array("文件MD5码验证错误") -> (w1339:string[])
                          n840 = call "表格编辑.vi"("新元素/子数组"=w1339, "活动单元格:单元格背景色"=u32 16711680, "MCListbox引用句柄"=w1338) -> ()  [unwired: 9 out]
                        }
                        frame True {
                        }
                      }
                    }
                  }
                  n841 = call <vilib>:"Unset Busy.vi"() -> ()  [unwired: 11 in, 1 out]
                }
                frame True {
                  n842 = stacked-sequence {
                    seq-local: [w1347 _ _ _] -> [_ w1575 w1669 _]
                    seq-local: [w1345 _ _ _] -> [_ w1553 _ _]
                    tunnel: w1342 -> [w1343 _ _ _]
                    tunnel: w1341 -> [w1360 _ _ w1696]
                    frame #0 {
